vi "NI VeriStand - Get Target Ref.vi"(8 "error in":errorcluster, 11 "Item Ref in":T1 format="%.0x") -> (0 "error out":errorcluster, 2 "Target Ref":T1 format="%.0x", 3 "Item Ref out":T1 format="%.0x", 4 "Found":bool)   [LabVIEW 2020, in "Custom Device Utility Library.lvlib"]
doc: "Gets a reference to the target on which the custom device that contains <B>Item Ref in</B> is running."
uses:
  <vilib>/NI VeriStand/Custom Device Tools/Custom Device Utility Library/Custom Device Utility Library.lvlib
  <vilib>/NI VeriStand/Custom Device API/Custom Device Item Ref.ctl
  <vilib>/NI VeriStand/Custom Device Tools/Custom Device Utility Library/NI VeriStand - Ref Constants.vi
  <vilib>/NI VeriStand/Custom Device API/Custom Device API.lvlib
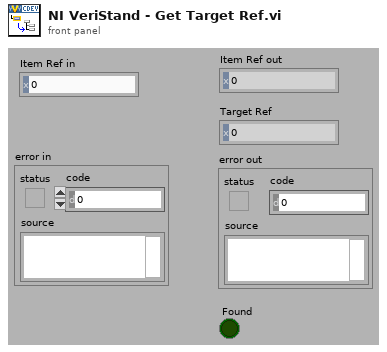
[diagram p1: front panel]
types:
  T1 = typedef "Custom Device API.lvlib/Custom Device Item Ref.ctl" = u64
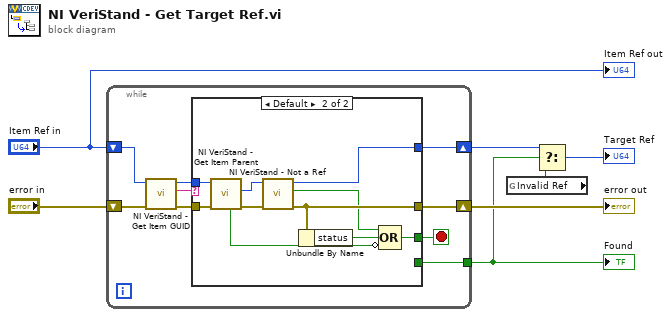
[diagram p0: block diagram]
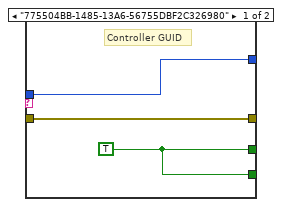
[diagram p2: hidden frame]
diagram:
  n1 = while {
    shift-right: [w11] -> w5
    shift-left: "error in" -> [w14]
    shift-right: [w10] -> w3
    shift-left: "Item Ref in" -> [w13]
    tunnel: [w8] -> w4
    stop <- w12 stop-if-true
    n2 = call <vilib>:"NI VeriStand - Get Item GUID.vi"("error in (no error)"=w14, "Item Ref in"=w13) -> ("error out"=w16:errorcluster, "GUID"=w9:string, "Item Ref out"=w15:T1)  [unwired: 7 out]
    n3 = case shown="Default" w9 {
      tunnel: w16 -> [w18 w29]
      tunnel: w15 -> [w19 w28]
      tunnel: [w17 w25] -> w12
      tunnel: [w18 w23] -> w11
      tunnel: [w19 w20] -> w10
      tunnel: [w17 _] -> w8
      frame "775504BB-1485-13A6-56755DBF2C326980" {
        w17 = TRUE
        # "Controller GUID"
      }
      frame Default {
        n4 = call <vilib>:"NI VeriStand - Get Item Parent.vi"("error in (no error)"=w29, "Item Ref in"=w28) -> ("error out"=w24:errorcluster, "Parent Ref"=w21:T1, "Found"=w26:bool)  [unwired: 7 out]
        n5 = call <vilib>:"NI VeriStand - Not a Ref.vi"("error in (no error)"=w24, "Item Ref"=w21) -> ("error out"=w23:errorcluster, "Not a Ref"=w22:bool, "Item Ref out"=w20:T1)  [unwired: 7 out]
        n6 = Unbundle By Name(w23) -> ("status"=w27:bool)
        n7 = Compound Arithmetic op=OR(w22, w27, invert w26) -> (w25:bool)
      }
    }
  }
  "Found" <- w4
  "error out" <- w5
  n8 = global read "NI VeriStand - Ref Constants.vi" "Invalid Ref"() -> (w1:T1)
  n9 = Select(t=w3, s=w4, f=w1) -> (s? t:f=→"Target Ref":T1)
  "Item Ref out" <- "Item Ref in"
